vi "Plot_selected_dataset.vi"(0 "selection":T2(ring), 1 "input xy data arrays":cluster{"all rows":dbl[][]}[](array[cluster]), 3 "file names and switch":T1(array[cluster])=[{"String"="nh4cucl.011", "Boolean"=TRUE, "begin"=9, "end"=9, "Numeric"=0.0}]) -> (2 "show files out":T1(array[cluster]), 4 "selected data set":string[](array[string]), 5 "default selection":T2(ring), 6 "selected xy data arrays":cluster{"all rows":dbl[][]}[](array[cluster]), 7 "selected elements":i32[](array[numeric]), 8 "selected files2":T3(array[cluster]), 9 "selected showfiles":T1(array[cluster]))   [LabVIEW 2024]
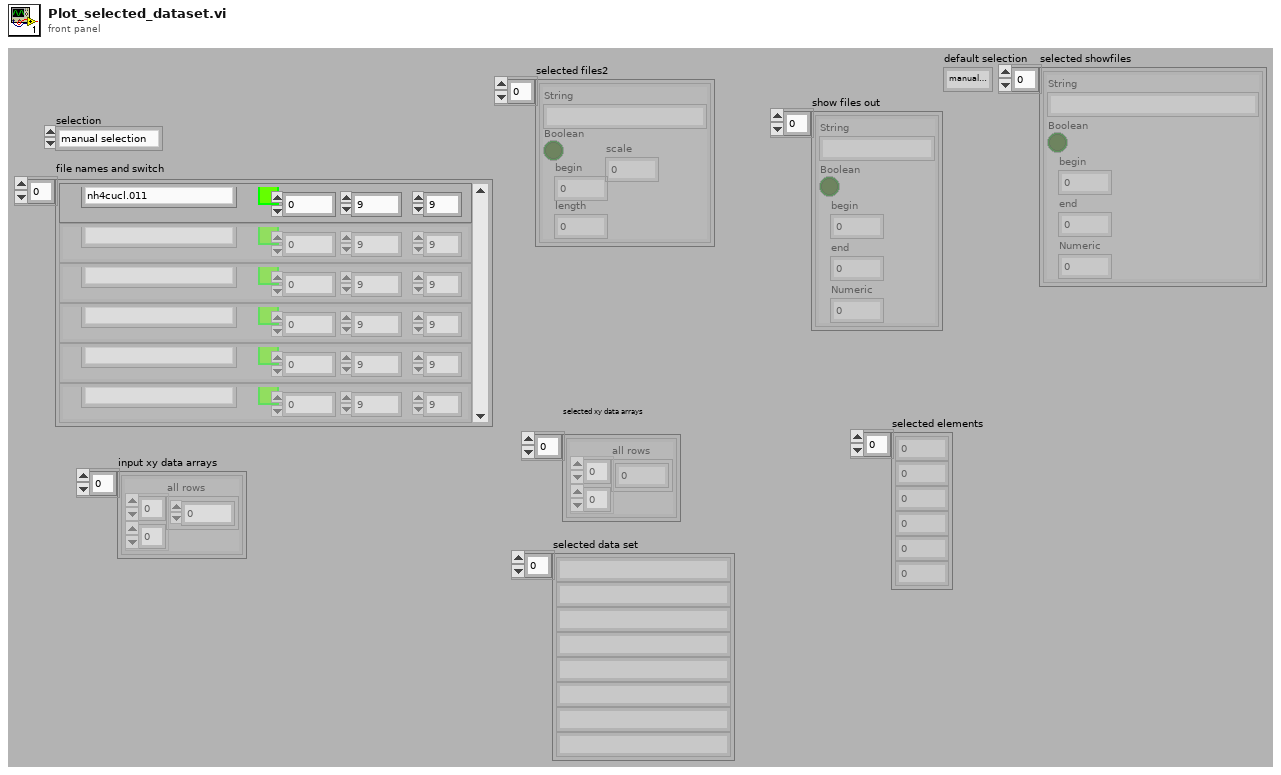
[diagram p1: front panel]
types:
  T1 = cluster{"String":string, "Boolean":bool, "begin":u32, "end":u32, "Numeric":dbl}[]
  T2 = enum16{"manual selection", "select all", "unselect all"}
  T3 = cluster{"String":string, "Boolean":bool, "begin":u32, "length":u32, "scale":dbl}[]
  T4 = cluster{"String":string, "Boolean":bool, "begin":u32, "end":u32, "Numeric":dbl}
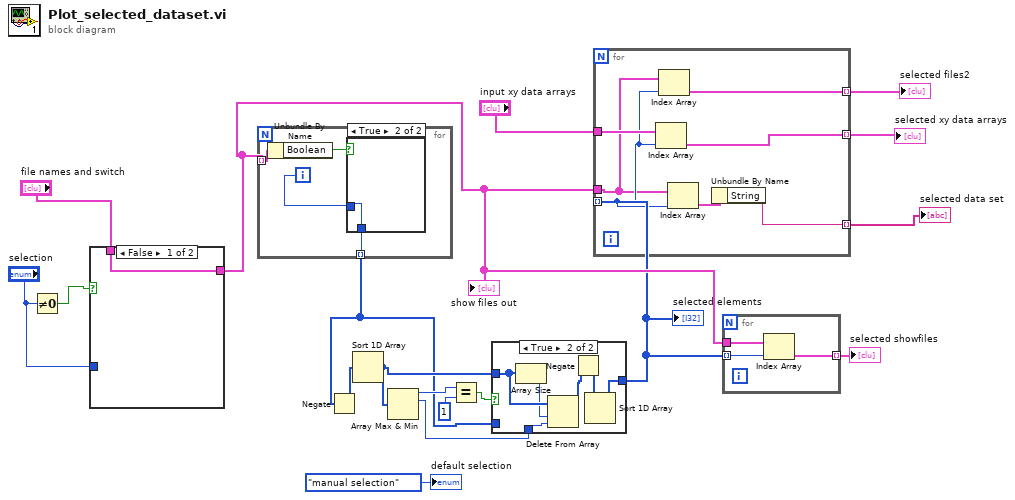
[diagram p0: block diagram]
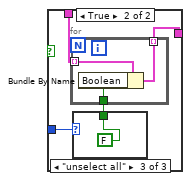
[diagram p2: hidden frame]
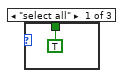
[diagram p3: hidden frame]
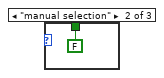
[diagram p4: hidden frame]
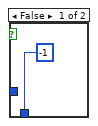
[diagram p6: hidden frame]
diagram:
  n1 = Not Equal To 0?(x="selection") -> (x != 0?=w6:bool)
  n2 = case shown="False" w6 {
    tunnel: "file names and switch" -> [w19 w23]
    tunnel: [w19 w22] -> w3
    tunnel: "selection" -> [_ w21]
    frame False {
    }
    frame True {
      n3 = case shown="\"unselect all\"" w21 {
        tunnel: [TRUE ("interpolate") FALSE ("interpolate") FALSE ("interpolate")] -> w20
        frame "select all" {
        }
        frame "manual selection" {
        }
        frame "unselect all" {
        }
      }
      n4 = for {
        tunnel: w23 -> [w29] mode=indexing
        tunnel: [w28] -> w22 mode=indexing
        tunnel: w20 -> [w27]
        n5 = Bundle By Name(cluster=w29, "Boolean"=w27) -> (w28:T4)
      }
    }
  }
  "show files out" <- w3
  n6 = for {
    tunnel: w3 -> [w33] mode=indexing
    tunnel: [w31] -> w12 mode=indexing
    i -> [w30]
    n7 = Unbundle By Name(w33) -> ("Boolean"=w32:bool)
    n8 = case shown="True" w32 {
      tunnel: w30 -> [_ w35]
      tunnel: [-1 w35] -> w31
      frame False {
      }
      frame True {
      }
    }
  }
  n9 = Negate(x=w12) -> (-x=w18:i32[])
  n10 = Sort 1D Array(array=w18) -> (sorted array=w17:i32[])
  n11 = Array Max & Min(array=w17) -> (max value=w13:i32, max index (indices)=w16:i32)  [unwired: 2 out]
  n12 = Equal?(x=w13, y=1) -> (x = y?=w15:bool)
  n13 = case shown="True" w15 {
    tunnel: w12 -> [w36 _]
    tunnel: [w36 w38] -> w2
    tunnel: w17 -> [_ w42]
    tunnel: w16 -> [_ w40]
    frame False {
    }
    frame True {
      n14 = Array Size(array=w42) -> (size(s)=w41:i32)
      n15 = Delete From Array(array=w42, length=w41, index=w40) -> (array with subset deleted=w39:i32[])  [unwired: 1 out]
      n16 = Negate(x=w39) -> (-x=w37:i32[])
      n17 = Sort 1D Array(array=w37) -> (sorted array=w38:i32[])
    }
  }
  "selected elements" <- w2
  n18 = for {
    tunnel: w2 -> [w45] mode=indexing
    tunnel: "input xy data arrays" -> [w49]
    tunnel: [w48] -> w10 mode=indexing
    tunnel: w3 -> [w44]
    tunnel: [w47] -> w9 mode=indexing
    tunnel: [w43] -> w8 mode=indexing
    n19 = Index Array(array=w49, index=w45) -> (element=w48:cluster{"all rows":dbl[][]})
    n20 = Index Array(array=w44, index=w45) -> (element=w43:T4)
    n21 = Index Array(array=w44, index=w45) -> (element=w46:T4)
    n22 = Unbundle By Name(w46) -> ("String"=w47:string)
  }
  "selected xy data arrays" <- w10
  "selected data set" <- w9
  "selected files2" <- w8
  n23 = for {
    tunnel: w3 -> [w52]
    tunnel: w2 -> [w51] mode=indexing
    tunnel: [w50] -> w1 mode=indexing
    n24 = Index Array(array=w52, index=w51) -> (element=w50:T4)
  }
  "selected showfiles" <- w1
  "default selection" <- T2."manual selection" ("selection")
